vi "Create X-Y channel lists.vi"(11 "Channels to plot":T1) -> (0 "Y names":string[](array[string]), 1 "Y-axis indexes":i32[](array[numeric]), 2 "X index":i32, 3 "X-axis name":string, 4 "Plots exist":bool)   [LabVIEW 2015]
uses:
  Utilities/Controls/Channels to plot.ctl
  Utilities/Controls/Channel to plot.ctl
panel:
  in  "Up Button":bool
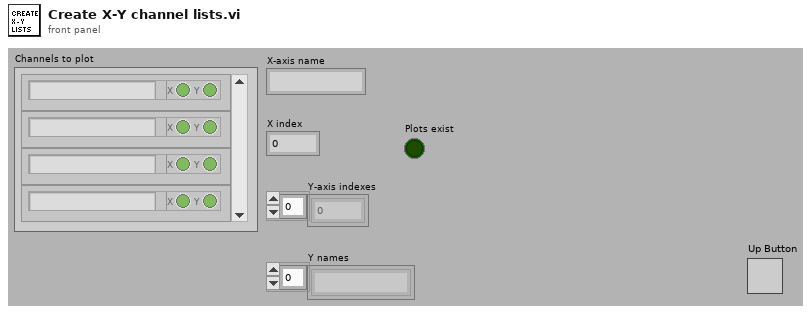
[diagram p1: front panel]
types:
  T1 = typedef "Channels to plot.ctl" = T2[]
  T2 = typedef "Channel to plot.ctl" = cluster{"Name":string, "X":bool, "Y":bool}
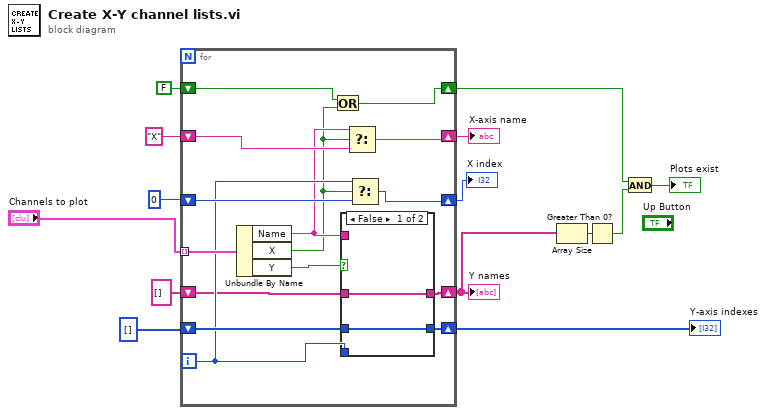
[diagram p0: block diagram]
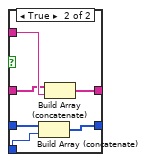
[diagram p2: hidden frame]
diagram:
  n1 = for {
    tunnel: "Channels to plot" -> [w22] mode=indexing
    shift-right: [w28] -> w13
    shift-left: i32[] [] -> [w27]
    shift-right: [w25] -> w14
    shift-left: 0 -> [w26]
    shift-right: [w23] -> w12
    shift-left: "X" -> [w24]
    shift-right: [w19] -> w5
    shift-left: string[] [] -> [w18]
    shift-right: [w16] -> w3
    shift-left: FALSE -> [w15]
    i -> [w21]
    n2 = Unbundle By Name(w22) -> ("Name"=w20:string, "X"=w17:bool, "Y"=w29:bool)
    n3 = Or(x=w15, y=w17) -> (x .or. y?=w16:bool)
    n4 = case shown="False" w29 {
      tunnel: [w31 w37] -> w28
      tunnel: w21 -> [_ w36]
      tunnel: w27 -> [w31 w35]
      tunnel: w20 -> [_ w34]
      tunnel: [w30 w33] -> w19
      tunnel: w18 -> [w30 w32]
      frame False {
      }
      frame True {
        n5 = Build Array (concatenate)(w35, w36) -> (w37:i32[])
        n6 = Build Array (concatenate)(w32, w34) -> (w33:string[])
      }
    }
    n7 = Select(t=w20, s=w17, f=w24) -> (s? t:f=w23:string)
    n8 = Select(t=w21, s=w17, f=w26) -> (s? t:f=w25:i32)
  }
  "X index" <- w14
  "Y-axis indexes" <- w13
  "Y names" <- w5
  "X-axis name" <- w12
  n9 = Array Size(array=w5) -> (size(s)=w6:i32)
  n10 = Greater Than 0?(x=w6) -> (x > 0?=w4:bool)
  n11 = And(x=w3, y=w4) -> (x .and. y?=→"Plots exist":bool)
